vi "findParentNodePath.vi"(8 "error in (no error)":errorcluster, 9 "nodePath":string, 10 "searchElement":string="channel_number type=\"analog\"", 11 "xmlNode in":refnum<class "xmlNode.lvclass">) -> (0 "error out":errorcluster, 2 "Paths":string[](array[string]), 3 "xmlNode out":refnum<class "xmlNode.lvclass">)   [LabVIEW 2009, in "Tools.lvlib" / "xml.lvlib" / "xmlNode.lvclass"]
uses:
  xmlNode.lvclass
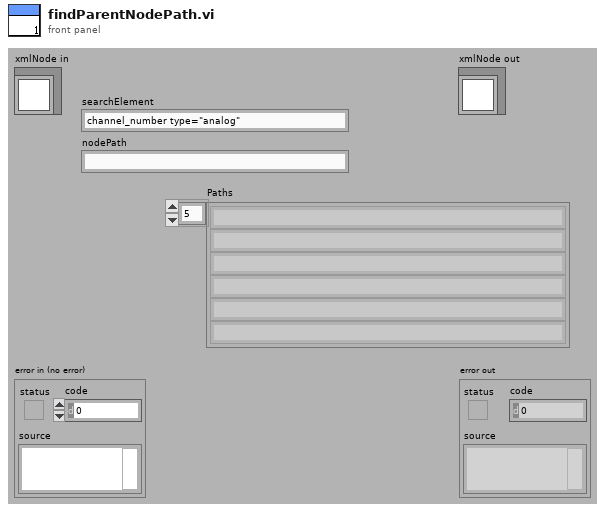
[diagram p1: front panel]
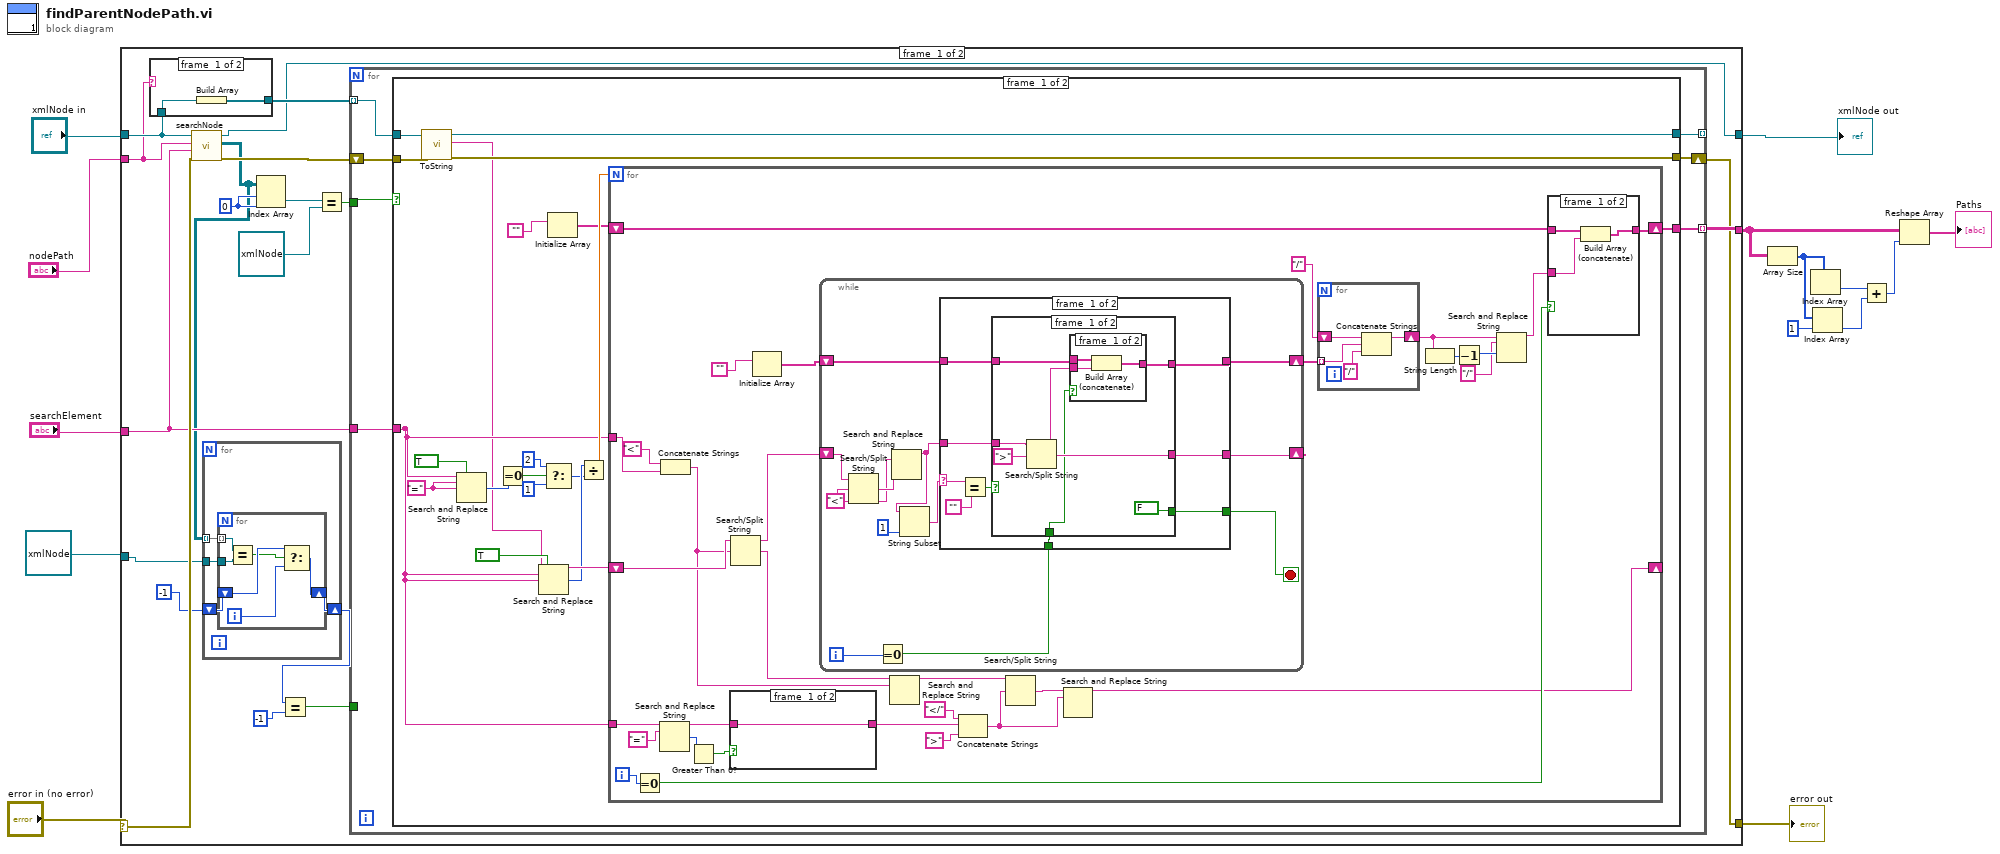
[diagram p0: block diagram]
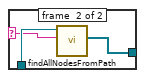
[diagram p2: hidden frame]
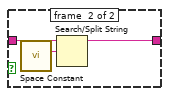
[diagram p3: hidden frame]
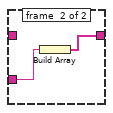
[diagram p4: hidden frame]
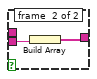
[diagram p5: hidden frame]
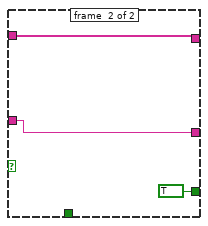
[diagram p6: hidden frame]
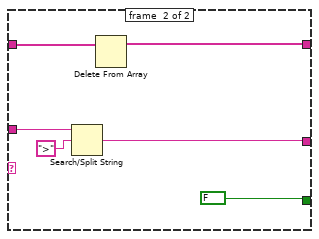
[diagram p7: hidden frame]
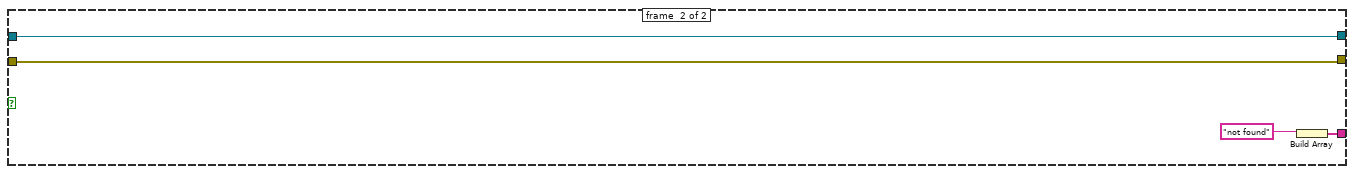
[diagram p8: hidden frame]
diagram:
  n1 = case shown="No Error" "error in (no error)" {
    selector: "error in (no error)" -> [w30 w167]
    tunnel: [w22 w167] -> w13
    tunnel: [w23 w168] -> w11
    tunnel: "xmlNode in" -> [w25 w168]
    tunnel: [w33 _] -> w4
    tunnel: "searchElement" -> [w29 _]
    tunnel: "nodePath" -> [w15 _]
    tunnel: refnum<class "xmlNode.lvclass"> refnum ("Tools.lvlib:xml.lvlib:xmlNode.lvclass") -> [w20 _]
    frame #0 {
      w27 = 0
      n2 = case shown="Default" w15 {
        selector: w15 -> [_ w36]
        tunnel: w25 -> [w35 w38]
        tunnel: [w34 w37] -> w24
        frame #0 {
          n3 = Build Array(w35) -> (w34:refnum<class "xmlNode.lvclass">[])
        }
        frame #1 {
          n4 = call "findAllNodesFromPath.vi"("nodePath"=w36, "xmlNode in"=w38) -> ("arrayXmlNodes"=w37:refnum<class "xmlNode.lvclass">[])  [unwired: 7 in, 2 out]
        }
      }
      n5 = call-dynamic "searchNode.vi"("error in (no error)"=w30, "searchElementName"=w29, "searchElementIn"=w15, "xmlNode in"=w25) -> ("error out"=w26:errorcluster, "arrayXmlNodes"=w21:refnum<class "xmlNode.lvclass">[][], "xmlNode out"=w23:refnum<class "xmlNode.lvclass">)  [unwired: 5 in]
      n6 = for {
        tunnel: w21 -> [w42] mode=indexing
        tunnel: w20 -> [w41]
        shift-right: [w39] -> w18
        shift-left: -1 -> [w40]
        n7 = for {
          tunnel: w42 -> [w47] mode=indexing
          tunnel: w41 -> [w48]
          shift-right: [w44] -> w39
          shift-left: w40 -> [w46]
          i -> [w45]
          n8 = Equal?(x=w47, y=w48) -> (x = y?=w43:bool)
          n9 = Select(t=w46, s=w43, f=w45) -> (s? t:f=w44:i32)
        }
      }
      n10 = Index Array(array=w21, index (row)=w27, index (col)=w27) -> (element=w32:refnum<class "xmlNode.lvclass">)
      n11 = Equal?(x=w18, y=-1) -> (x = y?=w16:bool)
      n12 = Equal?(x=w32, y=refnum<class "xmlNode.lvclass"> refnum ("Tools.lvlib:xml.lvlib:xmlNode.lvclass")) -> (x = y?=w28:bool)
      n13 = for {
        tunnel: [w55] -> w33 mode=indexing
        tunnel: w29 -> [w54]
        tunnel: w28 -> [w49]
        tunnel: [w53] -> _ mode=indexing
        tunnel: w24 -> [w51] mode=indexing
        shift-right: [w50] -> w22
        shift-left: w26 -> [w52]
        tunnel: w16 -> [_]
        n14 = case shown="False" w49 {
          tunnel: [w64 w166] -> w55
          tunnel: w54 -> [w63 _]
          tunnel: w51 -> [w62 w164]
          tunnel: [w61 w164] -> w53
          tunnel: w52 -> [w60 w163]
          tunnel: [w59 w163] -> w50
          frame #0 {
            w71 = "="
            n15 = call-dynamic "ToString.vi"("error in (no error)"=w60, "xmlNode in"=w62) -> ("error out"=w59:errorcluster, "xml"=w58:string, "xmlNode out"=w61:refnum<class "xmlNode.lvclass">)  [unwired: 7 in]
            n16 = Search and Replace String(replace all?=TRUE, input string=w63, search string=w71, replace string=w71) -> (number of replacements=w70:i32)  [unwired: 4 in, 3 out]
            n17 = Equal To 0?(x=w70) -> (x = 0?=w65:bool)
            n18 = Search and Replace String(replace all?=TRUE, input string=w58, search string=w63, replace string=w63) -> (result string=w74:string, number of replacements=w72:i32)  [unwired: 4 in, 2 out]
            n19 = Select(t=2, s=w65, f=1) -> (s? t:f=w68:i32)
            n20 = Initialize Array("") -> (w56:string[])  [unwired: 1 in]
            n21 = Divide(x=w72, y=w68) -> (x/y=w73:dbl)
            n22 = for {
              N: w73 -> [_]
              tunnel: w63 -> [w104]
              shift-right: [w83] -> _
              shift-left: w74 -> [w106]
              shift-right: [w96] -> w64
              shift-left: w56 -> [w95]
              tunnel: w63 -> [w90]
              i -> [w98]
              n23 = Equal To 0?(x=w98) -> (x = 0?=w97:bool)
              n24 = Search and Replace String(input string=w90, search string="=") -> (result string=w87:string, number of replacements=w89:i32)  [unwired: 6 in, 2 out]
              n25 = Concatenate Strings("<", w104) -> (w102:string)
              n26 = Greater Than 0?(x=w89) -> (x > 0?=w88:bool)
              n27 = case shown="True" w88 {
                tunnel: w87 -> [w107 w110]
                tunnel: [w107 w108] -> w86
                frame #0 {
                }
                frame #1 {
                  n28 = call <vilib>:"Space Constant.vi"() -> ("String"=w109:string)
                  n29 = Search/Split String(string=w110, search string/char (-)=w109) -> (substring before match=w108:string)  [unwired: 1 in, 2 out]
                }
              }
              n30 = Search/Split String(string=w106, search string/char (-)=w102) -> (substring before match=w101:string, match + rest of string=w103:string)  [unwired: 1 in, 1 out]
              n31 = Initialize Array("") -> (w76:string[])  [unwired: 1 in]
              n32 = while {
                shift-right: [w125] -> w100
                shift-left: w76 -> [w126]
                shift-right: [w128] -> _
                shift-left: w101 -> [w131]
                i -> [w127]
                stop <- w123 stop-if-true
                w121 = "<"
                n33 = Search/Split String(string=w131, search string/char (-)=w121) -> (match + rest of string=w122:string)  [unwired: 1 in, 2 out]
                n34 = Equal To 0?(x=w127) -> (x = 0?=w124:bool)
                n35 = Search and Replace String(input string=w122, search string=w121) -> (result string=w120:string)  [unwired: 6 in, 3 out]
                n36 = String Subset(string=w120, length (rest)=1) -> (substring=w130:string)  [unwired: 1 in]
                n37 = case shown="Default" w130 {
                  selector: w130 -> [w133 _]
                  tunnel: w120 -> [w140 w161]
                  tunnel: [w139 w159] -> w128
                  tunnel: [w137 w158] -> w125
                  tunnel: w126 -> [w138 w162]
                  tunnel: w124 -> [w136 _]
                  tunnel: [w135 FALSE] -> w123
                  frame #0 {
                    n38 = Equal?(x=w133, y="") -> (x = y?=w134:bool)
                    n39 = case shown="False" w134 {
                      tunnel: w140 -> [w148 w155]
                      tunnel: [w146 w155] -> w139
                      tunnel: w138 -> [w145 w156]
                      tunnel: [w144 w156] -> w137
                      tunnel: w136 -> [w142 _]
                      tunnel: [FALSE TRUE] -> w135
                      frame #0 {
                        n40 = Search/Split String(string=w148, search string/char (-)=">") -> (substring before match=w143:string, match + rest of string=w146:string)  [unwired: 1 in, 1 out]
                        n41 = case shown="True" w142 {
                          tunnel: w143 -> [w150 w152]
                          tunnel: w145 -> [w149 _]
                          tunnel: [w151 w153] -> w144
                          frame #0 {
                            n42 = Build Array (concatenate)(w149, w150) -> (w151:string[])
                          }
                          frame #1 {
                            n43 = Build Array(w152) -> (w153:string[])
                          }
                        }
                      }
                      frame #1 {
                      }
                    }
                  }
                  frame #1 {
                    n44 = Search/Split String(string=w161, search string/char (-)=">") -> (match + rest of string=w159:string)  [unwired: 1 in, 2 out]
                    n45 = Delete From Array(array=w162) -> (array with subset deleted=w158:string[])  [unwired: 2 in, 1 out]
                  }
                }
              }
              n46 = Search and Replace String(input string=w103, search string=w102) -> (result string=w94:string)  [unwired: 6 in, 3 out]
              n47 = Concatenate Strings("</", w86, ">") -> (w84:string)
              n48 = Search/Split String(string=w94, search string/char (-)=w84) -> (match + rest of string=w85:string)  [unwired: 1 in, 2 out]
              n49 = Search and Replace String(input string=w85, search string=w84) -> (result string=w83:string)  [unwired: 6 in, 3 out]
              n50 = for {
                tunnel: w100 -> [w118] mode=indexing
                shift-right: [w117] -> w79
                shift-left: "/" -> [w119]
                n51 = Concatenate Strings(w119, w118, "/") -> (w117:string)
              }
              n52 = String Length(string=w79) -> (length=w82:i32)
              n53 = Decrement(x=w82) -> (x-1=w81:i32)
              n54 = Search and Replace String(input string=w79, search string="/", offset=w81) -> (result string=w78:string)  [unwired: 5 in, 3 out]
              n55 = case shown="True" w97 {
                tunnel: w78 -> [w112 w115]
                tunnel: [w111 w114] -> w96
                tunnel: w95 -> [w113 _]
                frame #0 {
                  n56 = Build Array (concatenate)(w113, w112) -> (w111:string[])
                }
                frame #1 {
                  n57 = Build Array(w115) -> (w114:string[])
                }
              }
            }
          }
          frame #1 {
            n58 = Build Array("not found") -> (w166:string[])
          }
        }
      }
    }
    frame #1 {
    }
  }
  "error out" <- w13
  "xmlNode out" <- w11
  n59 = Array Size(array=w4) -> (size(s)=w8:i32[])
  n60 = Index Array(array=w8) -> (element=w6:i32)  [unwired: 1 in]
  n61 = Index Array(array=w8, index=1) -> (element=w5:i32)
  n62 = Add(x=w6, y=w5) -> (x+y=w3:i32)
  n63 = Reshape Array(w4, w3) -> (→"Paths":string[])
